vi "LSMcontroller_v63_3Dfocus.vi"() -> ()   [LabVIEW 2015] (continued)
                                w5034 = FALSE ("OK Button")
                                n2107 = property on="down" class="Bool (strict)"("Value"=w5034) -> ()  [unwired: 2 in, 2 out]
                                n2108 = property on="up" class="Bool (strict)"("Value"=w5034) -> ()  [unwired: 2 in, 2 out]
                                n2109 = property on="right" class="Bool (strict)"("Value"=w5034) -> ()  [unwired: 2 in, 2 out]
                                n2110 = property on="left" class="Bool (strict)"("Value"=w5034) -> ()  [unwired: 2 in, 2 out]
                                n2111 = property on="upleft" class="Bool (strict)"("Value"=w5033) -> ()  [unwired: 2 in, 2 out]
                                n2112 = property on="upright" class="Bool (strict)"("Value"=w5033) -> ()  [unwired: 2 in, 2 out]
                                n2113 = property on="downleft" class="Bool (strict)"("Value"=w5033) -> ()  [unwired: 2 in, 2 out]
                                n2114 = property on="downright" class="Bool (strict)"("Value"=w5033) -> ()  [unwired: 2 in, 2 out]
                                }
                                }
                                }
                                }
                                }
                              }
                              n2115 = dll-call lib="phlib.dll" fn="_PH_GetCountRate@8" label="PH_GetCountRate"("devidx"=w4980, "channel"=1) -> (→"Ch1Rate":i32)  [unwired: 5 in, 2 out]
                              n2116 = local read "Stop"() -> (w4982:bool)
                              n2117 = local write "points recorded"(w4979) -> ()
                            }
                          }
                          frame #3 {
                            w5042 = FALSE ("Value (Signaling)")
                            n2118 = call "2pparameters.vi"("command"="get") -> ("params out"=w5036:T10)  [unwired: 1 in]
                            n2119 = Unbundle By Name(w5036) -> ("autoshutter"=w5037:bool)
                            n2120 = case shown="True" w5037 {
                              frame False {
                              }
                              frame True {
                                n2121 = call "shuttercontrol.vi"("command"="close") -> ()  [unwired: 1 in, 1 out]
                              }
                            }
                            n2122 = property on="Start" class="Bool (strict)"("Val(Sgnl)"=w5042) -> ()  [unwired: 2 in, 2 out]
                            n2123 = property on="Start" class="Bool (strict)"("Visible"=TRUE, "DisabledEnum"=T7."Enabled" ("Disabled")) -> ()  [unwired: 2 in, 2 out]
                            n2124 = property on="Stop" class="Bool (strict)"("Val(Sgnl)"=w5042) -> ()  [unwired: 2 in, 2 out]
                            n2125 = property on="Stop" class="Bool (strict)"("Visible"=FALSE, "DisabledEnum"=T7."Disabled" ("Disabled")) -> ()  [unwired: 2 in, 2 out]
                          }
                        }
                      }
                      frame Enabled {
                      }
                    }
                    n2126 = local write "64bit disabled"(TRUE ("64bit disabled")) -> ()
                  }
                }
              }
            }
          }
          event "avpp", "Angle ref", "xpixels ref", "Vx-min ref", "Vx-max ref", "ypixels ref", "Vy-min ref", "Vy-max ref", "ROI Type", "Sampling rate": Value Change {
            n2127 = event-data() -> ()  [unwired: 1 in, 6 out]
            n2128 = local read "avpp"() -> (w5061:i32)
            n2129 = local read "Angle ref"() -> (w5060:dbl)
            n2130 = local read "ROI Type"() -> (w5059:u16)
            n2131 = local read "xpixels ref"() -> (w5056:i32)
            n2132 = local read "Vx-min ref"() -> (w5055:dbl)
            n2133 = local read "Vx-max ref"() -> (w5054:dbl)
            n2134 = local read "ypixels ref"() -> (w5052:i32)
            n2135 = local read "Vy-min ref"() -> (w5053:dbl)
            n2136 = local read "Vy-max ref"() -> (w5049:dbl)
            n2137 = local read "Sampling rate"() -> (w5044:dbl)
            n2138 = local read "# of frames"() -> (w5048:i32)
            n2139 = local read "maxbufferAI"() -> (w5047:i32)
            n2140 = local read "Override AI buffer"() -> (w5045:bool)
            n2141 = call "2pparameters.vi"("command"="get") -> ("params out"=w5058:T10)  [unwired: 1 in]
            n2142 = Bundle By Name(cluster=w5058, "avpp"=w5061, "Angle Img"=w5060, "Xpixels Img"=w5056, "Vx-min Img"=w5055, "VX-max Img"=w5054, "Ypixels Img"=w5052, "Vy-min Img"=w5053, "Vy-max Img"=w5049, "srate"=w5044, "srate Img"=w5044, "measpoints"=w5048, "maxbufferAI"=w5047, "Drawing Mode"=w5059, "Vz-reset"=0.0, "AIoverride"=w5045) -> (w5050:T10)
            n2143 = call "2pparameters.vi"("Params in"=w5050, "command"="set") -> ()  [unwired: 1 out]
          }
          event "# of frames": Value Change {
            n2144 = event-data() -> ()  [unwired: 1 in, 6 out]
            n2145 = local read "Meastab"() -> (w5062:enum32{"X-Y Image", "Linescan", "Timetrace"})
            n2146 = case shown="\"X-Y Image\", Default" w5062 {
              frame "X-Y Image", Default {
                n2147 = local read "# of frames"() -> (w5063:i32)
                n2148 = call "2pparameters.vi"("command"="get") -> ("params out"=w5067:T10)  [unwired: 1 in]
                n2149 = Bundle By Name(cluster=w5067, "measpoints"=w5063) -> (w5064:T10)
                n2150 = call "2pparameters.vi"("Params in"=w5064, "command"="set") -> ()  [unwired: 1 out]
              }
              frame "Linescan" {
                n2151 = local read "srateAODOtt"() -> (w5077:dbl)
                n2152 = local read "# of frames"() -> (w5073:i32)
                n2153 = local read "refreshtime"() -> (w5079:dbl)
                n2154 = local read "bin"() -> (w5074:dbl)
                n2155 = call "tt_timeandsamples.vi"("bin"=w5074, "refreshtime"=w5079, "srateAODOtt"=w5077, "tot#ofsamples"=w5073) -> ("refreshrate"=w5076:dbl, "refreshbuffer"=w5075:i32, "timetracecycles"=w5072:i32)  [unwired: 5 in]
                n2156 = call "2pparameters.vi"("command"="get") -> ("params out"=w5069:T10)  [unwired: 1 in]
                n2157 = Bundle By Name(cluster=w5069, "measpoints"=w5073, "tt_cycles"=w5072, "refreshbuffer"=w5075, "refreshrate"=w5076) -> (w5071:T10)
                n2158 = Reciprocal(x=w5076) -> (1/x=w5078:dbl)
                n2159 = local write "refreshtime"(w5078) -> ()
                n2160 = call "2pparameters.vi"("Params in"=w5071, "command"="set") -> ()  [unwired: 1 out]
              }
              frame "Timetrace" {
                n2161 = local read "srateAODOtt"() -> (w5089:dbl)
                n2162 = local read "# of frames"() -> (w5085:i32)
                n2163 = local read "refreshtime"() -> (w5091:dbl)
                n2164 = local read "bin"() -> (w5086:dbl)
                n2165 = call "tt_timeandsamples.vi"("bin"=w5086, "refreshtime"=w5091, "srateAODOtt"=w5089, "tot#ofsamples"=w5085) -> ("refreshrate"=w5088:dbl, "refreshbuffer"=w5087:i32, "timetracecycles"=w5084:i32)  [unwired: 5 in]
                n2166 = call "2pparameters.vi"("command"="get") -> ("params out"=w5081:T10)  [unwired: 1 in]
                n2167 = Bundle By Name(cluster=w5081, "measpoints"=w5085, "tt_cycles"=w5084, "refreshbuffer"=w5087, "refreshrate"=w5088) -> (w5083:T10)
                n2168 = Reciprocal(x=w5088) -> (1/x=w5090:dbl)
                n2169 = local write "refreshtime"(w5090) -> ()
                n2170 = call "2pparameters.vi"("Params in"=w5083, "command"="set") -> ()  [unwired: 1 out]
              }
            }
          }
          event "srateAODOtt", "refreshtime", "Vx-ref", "Vy-ref", "Vx-min draw", "Vx-max draw", "Vy-min draw", "Vy-max draw", "bin": Value Change {
            n2171 = event-data() -> ()  [unwired: 1 in, 6 out]
            n2172 = local read "ypixels ref"() -> (w5123:i32)
            n2173 = local read "Vy-min draw"() -> (w5099:dbl)
            n2174 = local read "Vy-max draw"() -> (w5098:dbl)
            n2175 = local read "Vx-min draw"() -> (w5101:dbl)
            n2176 = local read "Vx-max draw"() -> (w5100:dbl)
            n2177 = local read "xpixels ref"() -> (w5097:i32)
            n2178 = local read "ROI Type"() -> (w5096:u16)
            n2179 = local read "Pel"() -> (w5095:dbl)
            n2180 = local read "srateAODOtt"() -> (w5105:dbl)
            n2181 = local read "# of frames"() -> (w5110:i32)
            n2182 = local read "refreshtime"() -> (w5103:dbl)
            n2183 = local read "bin"() -> (w5108:dbl)
            n2184 = local read "Override AI buffer"() -> (w5093:bool)
            n2185 = local read "finite samples"() -> (w5117:bool)
            n2186 = local read "srateAODOtt"() -> (w5092:dbl)
            n2187 = local read "srateAODOtt"() -> (w5111:dbl)
            n2188 = local read "continuous"() -> (w5116:bool)
            n2189 = local read "Angle ref"() -> (w5102:dbl)
            n2190 = local read "wavdet"() -> (w5118:bool)
            n2191 = local read "Vx-ref"() -> (w5113:dbl)
            n2192 = local read "Vy-ref"() -> (w5115:dbl)
            n2193 = local read "avpp"() -> (w5114:i32)
            n2194 = call "tt_timeandsamples.vi"("bin"=w5108, "refreshtime"=w5103, "srateAODOtt"=w5105, "tot#ofsamples"=w5110) -> ("refreshrate"=w5106:dbl, "refreshbuffer"=w5107:i32, "timetracecycles"=w5112:i32)  [unwired: 5 in]
            n2195 = local read "bin"() -> (w5109:dbl)
            n2196 = call "2pparameters.vi"("command"="get") -> ("params out"=w5121:T10)  [unwired: 1 in]
            n2197 = Bundle By Name(cluster=w5121, "Drawing Mode"=w5096, "measpoints"=w5110, "tt_cycles"=w5112, "refreshbuffer"=w5107, "refreshrate"=w5106, "Vx-ref"=w5113, "Vy-ref"=w5115, "srate"=w5092, "finite"=w5117, "cont"=w5116, "wavdet"=w5118, "avpp"=w5114, "srateAODO"=w5111, "bufferAI"=w5107, "bin"=w5109, "Angle Img"=w5102, "Vxminref"=w5101, "Vxmaxref"=w5100, "Vyminref"=w5099, "Vymaxref"=w5098, "Xpixels Img"=w5097, "Ypixels Img"=w5123, "Pel"=w5095, "Vz-reset"=0.0, "AIoverride"=w5093) -> (w5119:T10)
            n2198 = Reciprocal(x=w5106) -> (1/x=w5104:dbl)
            n2199 = local write "refreshtime"(w5104) -> ()
            n2200 = call "2pparameters.vi"("Params in"=w5119, "command"="set") -> ()  [unwired: 1 out]
          }
          event "Init": Value Change {
            # "Disabled for conversion to 64 bit"
            n2201 = event-data() -> ()  [unwired: 1 in, 6 out]
            n2202 = disable-structure shown="Disabled" {
              frame Disabled {
                n2203 = flat-sequence {
                  frame #0 {
                    n2204 = local read "Measurement"() -> (w5125:T4)
                    n2205 = case shown="\"Lifetime (scan)\", \"Lifetime (contour)\"" w5125 {
                      frame "X-Y-t movie", Default {
                      }
                      frame "Lifetime (point)" {
                        n2206 = stacked-sequence {
                          frame #0 {
                            n2207 = call "initialize.vi"("mode"=0) -> ()
                          }
                          frame #1 {
                            n2208 = call "calib.vi"() -> ()  [unwired: 1 in]
                          }
                        }
                      }
                      frame "Lifetime (scan)", "Lifetime (contour)" {
                        n2209 = stacked-sequence {
                          frame #0 {
                            n2210 = call "initialize.vi"("mode"=3) -> ()
                          }
                          frame #1 {
                            n2211 = call "calib.vi"() -> ()  [unwired: 1 in]
                          }
                        }
                      }
                    }
                  }
                  frame #1 {
                    n2212 = property on="Start" class="Bool (strict)"("Visible"=TRUE, "DisabledEnum"=T7."Enabled" ("Disabled")) -> ()  [unwired: 2 in, 2 out]
                    n2213 = property on="Init" class="Bool (strict)"("Visible"=FALSE, "DisabledEnum"=T7."Disabled and Grayed Out" ("Disabled"), "Value"=FALSE ("Init")) -> ()  [unwired: 2 in, 2 out]
                  }
                }
              }
              frame Enabled {
              }
            }
            n2214 = local write "64bit disabled"(TRUE ("64bit disabled")) -> ()
          }
          event "Measurement": Value Change {
            n2215 = event-data() -> ()  [unwired: 1 in, 5 out]
            n2216 = case shown="\"X-Y-t movie\"" "Measurement" {
              frame "X-Y-t movie" {
                w5135 = T7."Disabled" ("Disabled")
                w5134 = FALSE ("Visible")
                n2217 = call "2pparameters.vi"("command"="get") -> ("params out"=w5145:T10)  [unwired: 1 in]
                n2218 = local write "graphtab"(T5."image" ("graphtab")) -> ()
                n2219 = local write "Save tab"(enum32{"withsave", "withoutsave"}."withsave" ("Save tab")) -> ()
                n2220 = Bundle By Name(cluster=w5145, "type"="X-Y-t movie") -> (w5143:T10)
                n2221 = call "2pparameters.vi"("Params in"=w5143, "command"="set") -> ()  [unwired: 1 out]
                n2222 = property on="refreshtime" class="DigNum (strict)"("Visible"=FALSE, "DisabledEnum"=T7."Disabled and Grayed Out" ("Disabled")) -> ()  [unwired: 2 in, 2 out]
                n2223 = property on="ttt" class="Enum (strict)"("Visible"=FALSE) -> ()  [unwired: 2 in, 2 out]
                n2224 = property on="# of frames" class="DigNum (strict)"("DisabledEnum"=T7."Enabled" ("Disabled"), "Caption.Text"="# of frames") -> ()  [unwired: 2 in, 2 out]
                n2225 = property on="continuous" class="Bool (strict)"("Visible"=TRUE, "DisabledEnum"=T7."Enabled" ("Disabled")) -> ()  [unwired: 2 in, 2 out]
                n2226 = property on="finite samples" class="Bool (strict)"("Visible"=TRUE, "DisabledEnum"=T7."Enabled" ("Disabled")) -> ()  [unwired: 2 in, 2 out]
                n2227 = property on="avpp" class="DigNum (strict)"("Visible"=TRUE, "DisabledEnum"=T7."Enabled" ("Disabled")) -> ()  [unwired: 2 in, 2 out]
                n2228 = property on="srateAODOtt" class="DigNum (strict)"("Visible"=FALSE, "DisabledEnum"=T7."Disabled" ("Disabled")) -> ()  [unwired: 2 in, 2 out]
                n2229 = local write "save\ndata"(TRUE ("save\ndata")) -> ()
                n2230 = property on="finite samples" class="Bool (strict)"("Val(Sgnl)"=TRUE ("continuous for display")) -> ()  [unwired: 2 in, 2 out]
                n2231 = property on="continuous" class="Bool (strict)"("Value"=FALSE ("continuous for display")) -> ()  [unwired: 2 in, 2 out]
                n2232 = property on="Current Average" class="DigNum (strict)"("Visible"=TRUE, "DisabledEnum"=T7."Enabled" ("Disabled")) -> ()  [unwired: 2 in, 2 out]
                n2233 = property on="img_CH1" class="IntGraph (strict)"("ZScale.Maximum"=7.0 ("Z Scale.Range:Maximum")) -> ()  [unwired: 2 in, 2 out]
                n2234 = property on="Sampling rate" class="DigNum (strict)"("Visible"=TRUE, "DisabledEnum"=T7."Enabled" ("Disabled")) -> ()  [unwired: 2 in, 2 out]
                n2235 = property on="Pel" class="DigNum (strict)"("Visible"=w5134, "DisabledEnum"=w5135) -> ()  [unwired: 2 in, 2 out]
                n2236 = property on="bin" class="DigNum (strict)"("Visible"=w5134, "DisabledEnum"=w5135) -> ()  [unwired: 2 in, 2 out]
                "Meastab" <- enum32{"X-Y Image", "Linescan", "Timetrace"}."X-Y Image" ("Meastab")
                "Zscantab" <- enum32{"withzscan", "withoutzscan", "lifetime"}."withoutzscan" ("Zscantab")
              }
              frame "X-Y-Z stack" {
                w5167 = T7."Disabled" ("Disabled")
                w5166 = FALSE ("Visible")
                n2237 = call "2pparameters.vi"("command"="get") -> ("params out"=w5177:T10)  [unwired: 1 in]
                n2238 = call "2pparameters.vi"("command"="get") -> ("params out"=w5181:T10)  [unwired: 1 in]
                n2239 = Bundle By Name(cluster=w5177, "type"="X-Y-Z stack") -> (w5175:T10)
                n2240 = Unbundle By Name(w5181) -> ("motorref"=w5180:refnum<k7>)
                n2241 = call "2pparameters.vi"("Params in"=w5175, "command"="set") -> ()  [unwired: 1 out]
                n2242 = local write "Zscantab"(enum32{"withzscan", "withoutzscan", "lifetime"}."withzscan" ("Zscantab")) -> ()
                n2243 = local write "Meastab"(enum32{"X-Y Image", "Linescan", "Timetrace"}."X-Y Image" ("Meastab")) -> ()
                n2244 = invoke class="MG17Motor" method="GetPosition"(reference=w5180, "lChanID"=0, "pfPosition"=sgl 0.0) -> ("pfPosition"=w5192:sgl)  [unwired: 2 in, 4 out]
                n2245 = property on="refreshtime" class="DigNum (strict)"("Visible"=FALSE, "DisabledEnum"=T7."Disabled and Grayed Out" ("Disabled")) -> ()  [unwired: 2 in, 2 out]
                n2246 = property on="ttt" class="Enum (strict)"("Visible"=FALSE) -> ()  [unwired: 2 in, 2 out]
                n2247 = Multiply(x=w5192, y=1000.0) -> (x*y=w5191:dbl)
                n2248 = local write "Actual Z position"(w5191) -> ()
                n2249 = local write "Save tab"(enum32{"withsave", "withoutsave"}."withsave" ("Save tab")) -> ()
                n2250 = property on="finite samples" class="Bool (strict)"("Visible"=FALSE, "DisabledEnum"=T7."Disabled and Grayed Out" ("Disabled")) -> ()  [unwired: 2 in, 2 out]
                n2251 = property on="avpp" class="DigNum (strict)"("Visible"=TRUE, "DisabledEnum"=T7."Enabled" ("Disabled")) -> ()  [unwired: 2 in, 2 out]
                n2252 = property on="continuous" class="Bool (strict)"("Visible"=FALSE, "DisabledEnum"=T7."Disabled and Grayed Out" ("Disabled")) -> ()  [unwired: 2 in, 2 out]
                n2253 = property on="img_CH1" class="IntGraph (strict)"("ZScale.Maximum"=7.0 ("Z Scale.Range:Maximum")) -> ()  [unwired: 2 in, 2 out]
                n2254 = property on="srateAODOtt" class="DigNum (strict)"("Visible"=FALSE, "DisabledEnum"=T7."Disabled" ("Disabled")) -> ()  [unwired: 2 in, 2 out]
                n2255 = property on="Pel" class="DigNum (strict)"("Visible"=w5166, "DisabledEnum"=w5167) -> ()  [unwired: 2 in, 2 out]
                n2256 = property on="bin" class="DigNum (strict)"("Visible"=w5166, "DisabledEnum"=w5167) -> ()  [unwired: 2 in, 2 out]
                n2257 = property on="Current Average" class="DigNum (strict)"("Visible"=TRUE, "DisabledEnum"=T7."Enabled" ("Disabled")) -> ()  [unwired: 2 in, 2 out]
                n2258 = property on="# of frames" class="DigNum (strict)"("Caption.Text"="# of slices", "DisabledEnum"=T7."Disabled and Grayed Out" ("Disabled")) -> ()  [unwired: 2 in, 2 out]
                n2259 = local write "save\ndata"(TRUE ("save\ndata")) -> ()
                n2260 = property on="finite samples" class="Bool (strict)"("Val(Sgnl)"=TRUE ("continuous for display")) -> ()  [unwired: 2 in, 2 out]
                n2261 = property on="continuous" class="Bool (strict)"("Value"=FALSE ("continuous for display")) -> ()  [unwired: 2 in, 2 out]
                n2262 = property on="Sampling rate" class="DigNum (strict)"("Visible"=TRUE, "DisabledEnum"=T7."Enabled" ("Disabled")) -> ()  [unwired: 2 in, 2 out]
              }
              frame "X-Y-Z-t movie" {
                w5206 = T7."Disabled" ("Disabled")
                w5205 = FALSE ("Visible")
                n2263 = property on="# of frames" class="DigNum (strict)"("DisabledEnum"=T7."Enabled" ("Disabled")) -> ()  [unwired: 2 in, 2 out]
                n2264 = property on="Current Average" class="DigNum (strict)"("Visible"=TRUE, "DisabledEnum"=T7."Enabled" ("Disabled")) -> ()  [unwired: 2 in, 2 out]
                n2265 = property on="avpp" class="DigNum (strict)"("Visible"=TRUE, "DisabledEnum"=T7."Enabled" ("Disabled")) -> ()  [unwired: 2 in, 2 out]
                n2266 = local write "Save tab"(enum32{"withsave", "withoutsave"}."withsave" ("Save tab")) -> ()
                n2267 = local write "Zscantab"(enum32{"withzscan", "withoutzscan", "lifetime"}."withzscan" ("Zscantab")) -> ()
                n2268 = local write "Meastab"(enum32{"X-Y Image", "Linescan", "Timetrace"}."X-Y Image" ("Meastab")) -> ()
                n2269 = property on="refreshtime" class="DigNum (strict)"("Visible"=FALSE, "DisabledEnum"=T7."Disabled and Grayed Out" ("Disabled")) -> ()  [unwired: 2 in, 2 out]
                n2270 = property on="ttt" class="Enum (strict)"("Visible"=FALSE) -> ()  [unwired: 2 in, 2 out]
                n2271 = call "2pparameters.vi"("command"="get") -> ("params out"=w5216:T10)  [unwired: 1 in]
                n2272 = Bundle By Name(cluster=w5216, "type"="X-Y-Z-t movie") -> (w5214:T10)
                n2273 = property on="continuous" class="Bool (strict)"("Visible"=TRUE, "DisabledEnum"=T7."Enabled" ("Disabled")) -> ()  [unwired: 2 in, 2 out]
                n2274 = property on="finite samples" class="Bool (strict)"("Visible"=TRUE, "DisabledEnum"=T7."Enabled" ("Disabled")) -> ()  [unwired: 2 in, 2 out]
                n2275 = call "2pparameters.vi"("Params in"=w5214, "command"="set") -> ()  [unwired: 1 out]
                n2276 = property on="srateAODOtt" class="DigNum (strict)"("Visible"=FALSE, "DisabledEnum"=T7."Disabled" ("Disabled")) -> ()  [unwired: 2 in, 2 out]
                n2277 = local write "save\ndata"(TRUE ("save\ndata")) -> ()
                n2278 = property on="img_CH1" class="IntGraph (strict)"("ZScale.Maximum"=7.0 ("Z Scale.Range:Maximum")) -> ()  [unwired: 2 in, 2 out]
                n2279 = property on="continuous" class="Bool (strict)"("Value"=FALSE ("continuous for display")) -> ()  [unwired: 2 in, 2 out]
                n2280 = property on="finite samples" class="Bool (strict)"("Value"=TRUE ("continuous for display")) -> ()  [unwired: 2 in, 2 out]
                n2281 = property on="Sampling rate" class="DigNum (strict)"("Visible"=TRUE, "DisabledEnum"=T7."Enabled" ("Disabled")) -> ()  [unwired: 2 in, 2 out]
                n2282 = property on="Pel" class="DigNum (strict)"("Visible"=w5205, "DisabledEnum"=w5206) -> ()  [unwired: 2 in, 2 out]
                n2283 = property on="bin" class="DigNum (strict)"("Visible"=w5205, "DisabledEnum"=w5206) -> ()  [unwired: 2 in, 2 out]
              }
              frame "linescan" {
                w5236 = T7."Enabled" ("Disabled")
                w5235 = TRUE ("Visible")
                w5238 = T7."Enabled" ("Disabled")
                w5237 = TRUE ("Visible")
                n2284 = local write "Meastab"(enum32{"X-Y Image", "Linescan", "Timetrace"}."Linescan" ("Meastab")) -> ()
                n2285 = property on="Current Average" class="DigNum (strict)"("Visible"=TRUE, "DisabledEnum"=T7."Enabled" ("Disabled")) -> ()  [unwired: 2 in, 2 out]
                n2286 = local write "Save tab"(enum32{"withsave", "withoutsave"}."withsave" ("Save tab")) -> ()
                n2287 = local write "Zscantab"(enum32{"withzscan", "withoutzscan", "lifetime"}."withoutzscan" ("Zscantab")) -> ()
                n2288 = property on="refreshtime" class="DigNum (strict)"("Visible"=FALSE, "DisabledEnum"=T7."Disabled and Grayed Out" ("Disabled")) -> ()  [unwired: 2 in, 2 out]
                n2289 = property on="continuous" class="Bool (strict)"("Value"=FALSE ("continuous for display")) -> ()  [unwired: 2 in, 2 out]
                n2290 = property on="finite samples" class="Bool (strict)"("Value"=TRUE ("continuous for display")) -> ()  [unwired: 2 in, 2 out]
                n2291 = property on="ttt" class="Enum (strict)"("Visible"=FALSE) -> ()  [unwired: 2 in, 2 out]
                n2292 = local write "save\ndata"(TRUE ("save\ndata")) -> ()
                n2293 = call "2pparameters.vi"("command"="get") -> ("params out"=w5247:T10)  [unwired: 1 in]
                n2294 = Bundle By Name(cluster=w5247, "type"="linescan") -> (w5245:T10)
                n2295 = property on="# of frames" class="DigNum (strict)"("DisabledEnum"=T7."Enabled" ("Disabled"), "Caption.Text"="# of lines") -> ()  [unwired: 2 in, 2 out]
                n2296 = property on="continuous" class="Bool (strict)"("Visible"=TRUE, "DisabledEnum"=T7."Enabled" ("Disabled")) -> ()  [unwired: 2 in, 2 out]
                n2297 = property on="avpp" class="DigNum (strict)"("Visible"=TRUE, "DisabledEnum"=T7."Enabled" ("Disabled")) -> ()  [unwired: 2 in, 2 out]
                n2298 = property on="finite samples" class="Bool (strict)"("Visible"=TRUE, "DisabledEnum"=T7."Enabled" ("Disabled")) -> ()  [unwired: 2 in, 2 out]
                n2299 = property on="srateAODOtt" class="DigNum (strict)"("Visible"=TRUE, "DisabledEnum"=T7."Enabled" ("Disabled")) -> ()  [unwired: 2 in, 2 out]
                n2300 = call "2pparameters.vi"("Params in"=w5245, "command"="set") -> ()  [unwired: 1 out]
                n2301 = property on="Pel" class="DigNum (strict)"("Visible"=w5237, "DisabledEnum"=w5238) -> ()  [unwired: 2 in, 2 out]
                n2302 = property on="bin" class="DigNum (strict)"("Visible"=w5237, "DisabledEnum"=w5238) -> ()  [unwired: 2 in, 2 out]
                n2303 = property on="Sampling rate" class="DigNum (strict)"("Visible"=FALSE, "DisabledEnum"=T7."Disabled" ("Disabled")) -> ()  [unwired: 2 in, 2 out]
                n2304 = property on="Pel" class="DigNum (strict)"("Visible"=w5235, "DisabledEnum"=w5236) -> ()  [unwired: 2 in, 2 out]
                n2305 = property on="bin" class="DigNum (strict)"("Visible"=w5235, "DisabledEnum"=w5236) -> ()  [unwired: 2 in, 2 out]
              }
              frame "Timetrace" {
                w5268 = T7."Enabled" ("Disabled")
                w5267 = TRUE ("Visible")
                n2306 = call "2pparameters.vi"("command"="get") -> ("params out"=w5273:T10)  [unwired: 1 in]
                n2307 = local write "Meastab"(enum32{"X-Y Image", "Linescan", "Timetrace"}."Timetrace" ("Meastab")) -> ()
                n2308 = Unbundle By Name(w5273) -> ("Angle draw"=w5275:dbl)
                n2309 = local write "Zscantab"(enum32{"withzscan", "withoutzscan", "lifetime"}."withoutzscan" ("Zscantab")) -> ()
                n2310 = property on="# of frames" class="DigNum (strict)"("DisabledEnum"=T7."Enabled" ("Disabled"), "Caption.Text"="# of samples") -> ()  [unwired: 2 in, 2 out]
                n2311 = property on="refreshtime" class="DigNum (strict)"("Visible"=TRUE, "DisabledEnum"=T7."Enabled" ("Disabled")) -> ()  [unwired: 2 in, 2 out]
                n2312 = property on="avpp" class="DigNum (strict)"("Visible"=FALSE, "DisabledEnum"=T7."Disabled and Grayed Out" ("Disabled")) -> ()  [unwired: 2 in, 2 out]
                n2313 = property on="Current Average" class="DigNum (strict)"("Visible"=FALSE, "DisabledEnum"=T7."Disabled and Grayed Out" ("Disabled")) -> ()  [unwired: 2 in, 2 out]
                n2314 = local write "Angle drawing"(w5275) -> ()
                n2315 = property on="ttt" class="Enum (strict)"("Visible"=TRUE) -> ()  [unwired: 2 in, 2 out]
                n2316 = property on="continuous" class="Bool (strict)"("Visible"=TRUE, "DisabledEnum"=T7."Enabled" ("Disabled")) -> ()  [unwired: 2 in, 2 out]
                n2317 = property on="finite samples" class="Bool (strict)"("Visible"=TRUE, "DisabledEnum"=T7."Enabled" ("Disabled")) -> ()  [unwired: 2 in, 2 out]
                n2318 = local write "save\ndata"(TRUE ("save\ndata")) -> ()
                n2319 = property on="finite samples" class="Bool (strict)"("Val(Sgnl)"=TRUE ("continuous for display")) -> ()  [unwired: 2 in, 2 out]
                n2320 = property on="continuous" class="Bool (strict)"("Value"=FALSE ("continuous for display")) -> ()  [unwired: 2 in, 2 out]
                n2321 = local write "Save tab"(enum32{"withsave", "withoutsave"}."withsave" ("Save tab")) -> ()
                n2322 = property on="srateAODOtt" class="DigNum (strict)"("Visible"=TRUE, "DisabledEnum"=T7."Enabled" ("Disabled")) -> ()  [unwired: 2 in, 2 out]
                n2323 = call "2pparameters.vi"("command"="get") -> ("params out"=w5280:T10)  [unwired: 1 in]
                n2324 = Bundle By Name(cluster=w5280, "type"="Timetrace") -> (w5278:T10)
                n2325 = property on="Sampling rate" class="DigNum (strict)"("Visible"=FALSE, "DisabledEnum"=T7."Disabled" ("Disabled")) -> ()  [unwired: 2 in, 2 out]
                n2326 = property on="Pel" class="DigNum (strict)"("Visible"=w5267, "DisabledEnum"=w5268) -> ()  [unwired: 2 in, 2 out]
                n2327 = property on="bin" class="DigNum (strict)"("Visible"=w5267, "DisabledEnum"=w5268) -> ()  [unwired: 2 in, 2 out]
                n2328 = call "2pparameters.vi"("Params in"=w5278, "command"="set") -> ()  [unwired: 1 out]
              }
              frame "Lifetime (point)" {
                w5301 = T7."Enabled" ("Disabled")
                w5300 = TRUE ("Visible")
                n2329 = property on="Pel" class="DigNum (strict)"("Visible"=w5300, "DisabledEnum"=w5301) -> ()  [unwired: 2 in, 2 out]
                n2330 = property on="bin" class="DigNum (strict)"("Visible"=w5300, "DisabledEnum"=w5301) -> ()  [unwired: 2 in, 2 out]
                n2331 = property on="ttt" class="Enum (strict)"("Visible"=FALSE) -> ()  [unwired: 2 in, 2 out]
                n2332 = local write "Zscantab"(enum32{"withzscan", "withoutzscan", "lifetime"}."lifetime" ("Zscantab")) -> ()
                n2333 = local write "graphtab"(T5."Lifetime" ("graphtab")) -> ()
                n2334 = local write "Meastab"(enum32{"X-Y Image", "Linescan", "Timetrace"}."Timetrace" ("Meastab")) -> ()
                n2335 = call "lifetimeparameters.vi"("command"="get") -> ("Params out"=w5308:T19)  [unwired: 1 in]
                n2336 = Unbundle By Name(w5308) -> ("initialized"=w5309:bool)
                n2337 = property on="srateAODOtt" class="DigNum (strict)"("Visible"=TRUE, "DisabledEnum"=T7."Enabled" ("Disabled")) -> ()  [unwired: 2 in, 2 out]
                n2338 = case shown="False" w5309 {
                  frame False {
                    n2339 = property on="Init" class="Bool (strict)"("Visible"=TRUE, "DisabledEnum"=T7."Enabled" ("Disabled")) -> ()  [unwired: 2 in, 2 out]
                    n2340 = property on="Start" class="Bool (strict)"("Visible"=FALSE, "DisabledEnum"=T7."Disabled and Grayed Out" ("Disabled")) -> ()  [unwired: 2 in, 2 out]
                  }
                  frame True {
                  }
                }
                n2341 = property on="Sampling rate" class="DigNum (strict)"("Visible"=FALSE, "DisabledEnum"=T7."Disabled" ("Disabled")) -> ()  [unwired: 2 in, 2 out]
              }
              frame "Lifetime (scan)" {
                w5318 = T7."Disabled" ("Disabled")
                w5317 = FALSE ("Visible")
                n2342 = call "lifetimeparameters.vi"("command"="get") -> ("Params out"=w5330:T19)  [unwired: 1 in]
                n2343 = local write "graphtab"(T5."image" ("graphtab")) -> ()
                n2344 = local write "Save tab"(enum32{"withsave", "withoutsave"}."withsave" ("Save tab")) -> ()
                n2345 = local write "Meastab"(enum32{"X-Y Image", "Linescan", "Timetrace"}."X-Y Image" ("Meastab")) -> ()
                n2346 = local write "Zscantab"(enum32{"withzscan", "withoutzscan", "lifetime"}."lifetime" ("Zscantab")) -> ()
                n2347 = Unbundle By Name(w5330) -> ("initialized"=w5329:bool)
                n2348 = property on="ttt" class="Enum (strict)"("Visible"=FALSE) -> ()  [unwired: 2 in, 2 out]
                n2349 = property on="refreshtime" class="DigNum (strict)"("Visible"=FALSE, "DisabledEnum"=T7."Disabled and Grayed Out" ("Disabled")) -> ()  [unwired: 2 in, 2 out]
                n2350 = property on="Pel" class="DigNum (strict)"("Visible"=w5317, "DisabledEnum"=w5318) -> ()  [unwired: 2 in, 2 out]
                n2351 = property on="bin" class="DigNum (strict)"("Visible"=w5317, "DisabledEnum"=w5318) -> ()  [unwired: 2 in, 2 out]
                n2352 = property on="save data" class="Bool (strict)"("Visible"=TRUE, "DisabledEnum"=T7."Enabled" ("Disabled"), "Value"=TRUE ("Visible")) -> ()  [unwired: 2 in, 2 out]
                n2353 = case shown="False" w5329 {
                  frame False {
                    n2354 = property on="Init" class="Bool (strict)"("Visible"=TRUE, "DisabledEnum"=T7."Enabled" ("Disabled")) -> ()  [unwired: 2 in, 2 out]
                    n2355 = property on="Start" class="Bool (strict)"("Visible"=FALSE, "DisabledEnum"=T7."Disabled and Grayed Out" ("Disabled")) -> ()  [unwired: 2 in, 2 out]
                  }
                  frame True {
                  }
                }
                n2356 = call "2pparameters.vi"("command"="get") -> ("params out"=w5335:T10)  [unwired: 1 in]
                n2357 = property on="continuous" class="Bool (strict)"("Visible"=TRUE, "DisabledEnum"=T7."Disabled and Grayed Out" ("Disabled")) -> ()  [unwired: 2 in, 2 out]
                n2358 = property on="finite samples" class="Bool (strict)"("Visible"=TRUE, "DisabledEnum"=T7."Enabled" ("Disabled")) -> ()  [unwired: 2 in, 2 out]
                n2359 = Bundle By Name(cluster=w5335, "type"="Lifetime (scan)") -> (w5333:T10)
                n2360 = call "2pparameters.vi"("Params in"=w5333, "command"="set") -> ()  [unwired: 1 out]
                n2361 = property on="finite samples" class="Bool (strict)"("Val(Sgnl)"=TRUE ("continuous for display")) -> ()  [unwired: 2 in, 2 out]
                n2362 = property on="continuous" class="Bool (strict)"("Value"=FALSE ("continuous for display")) -> ()  [unwired: 2 in, 2 out]
                n2363 = property on="srateAODOtt" class="DigNum (strict)"("Visible"=FALSE, "DisabledEnum"=T7."Disabled" ("Disabled")) -> ()  [unwired: 2 in, 2 out]
                n2364 = property on="# of frames" class="DigNum (strict)"("DisabledEnum"=T7."Enabled" ("Disabled"), "Caption.Text"="# of frames") -> ()  [unwired: 2 in, 2 out]
                n2365 = property on="img_CH1" class="IntGraph (strict)"("ZScale.Maximum"=12.5 ("Z Scale.Range:Maximum")) -> ()  [unwired: 2 in, 2 out]
                n2366 = property on="Current Average" class="DigNum (strict)"("Visible"=TRUE, "DisabledEnum"=T7."Enabled" ("Disabled")) -> ()  [unwired: 2 in, 2 out]
                n2367 = property on="Sampling rate" class="DigNum (strict)"("Visible"=TRUE, "DisabledEnum"=T7."Enabled" ("Disabled")) -> ()  [unwired: 2 in, 2 out]
                n2368 = property on="avpp" class="DigNum (strict)"("Visible"=TRUE, "DisabledEnum"=T7."Enabled" ("Disabled")) -> ()  [unwired: 2 in, 2 out]
              }
              frame "Lifetime (contour)" {
                w5359 = T7."Enabled" ("Disabled")
                w5358 = TRUE ("Visible")
                n2369 = call "2pparameters.vi"("command"="get") -> ("params out"=w5366:T10)  [unwired: 1 in]
                n2370 = property on="# of frames" class="DigNum (strict)"("DisabledEnum"=T7."Enabled" ("Disabled"), "Caption.Text"="# of samples") -> ()  [unwired: 2 in, 2 out]
                n2371 = property on="refreshtime" class="DigNum (strict)"("Visible"=TRUE, "DisabledEnum"=T7."Enabled" ("Disabled")) -> ()  [unwired: 2 in, 2 out]
                n2372 = Unbundle By Name(w5366) -> ("Angle draw"=w5368:dbl)
                n2373 = property on="avpp" class="DigNum (strict)"("Visible"=FALSE, "DisabledEnum"=T7."Disabled and Grayed Out" ("Disabled")) -> ()  [unwired: 2 in, 2 out]
                n2374 = property on="Current Average" class="DigNum (strict)"("Visible"=FALSE, "DisabledEnum"=T7."Disabled and Grayed Out" ("Disabled")) -> ()  [unwired: 2 in, 2 out]
                n2375 = local write "Angle drawing"(w5368) -> ()
                n2376 = local write "Save tab"(enum32{"withsave", "withoutsave"}."withsave" ("Save tab")) -> ()
                n2377 = local write "Zscantab"(enum32{"withzscan", "withoutzscan", "lifetime"}."lifetime" ("Zscantab")) -> ()
                n2378 = local write "graphtab"(T5."Lifetime" ("graphtab")) -> ()
                n2379 = local write "Meastab"(enum32{"X-Y Image", "Linescan", "Timetrace"}."Timetrace" ("Meastab")) -> ()
                n2380 = property on="ttt" class="Enum (strict)"("Visible"=TRUE) -> ()  [unwired: 2 in, 2 out]
                n2381 = call "lifetimeparameters.vi"("command"="get") -> ("Params out"=w5390:T19)  [unwired: 1 in]
                n2382 = property on="finite samples" class="Bool (strict)"("Val(Sgnl)"=TRUE ("continuous for display")) -> ()  [unwired: 2 in, 2 out]
                n2383 = local write "save\ndata"(TRUE ("save\ndata")) -> ()
                n2384 = Unbundle By Name(w5390) -> ("initialized"=w5391:bool)
                n2385 = property on="continuous" class="Bool (strict)"("Visible"=TRUE, "DisabledEnum"=T7."Enabled" ("Disabled")) -> ()  [unwired: 2 in, 2 out]
                n2386 = property on="finite samples" class="Bool (strict)"("Visible"=TRUE, "DisabledEnum"=T7."Enabled" ("Disabled")) -> ()  [unwired: 2 in, 2 out]
                n2387 = property on="Pel" class="DigNum (strict)"("Visible"=w5358, "DisabledEnum"=w5359) -> ()  [unwired: 2 in, 2 out]
                n2388 = property on="bin" class="DigNum (strict)"("Visible"=w5358, "DisabledEnum"=w5359) -> ()  [unwired: 2 in, 2 out]
                n2389 = property on="continuous" class="Bool (strict)"("Value"=FALSE ("continuous for display")) -> ()  [unwired: 2 in, 2 out]
                n2390 = case shown="False" w5391 {
                  frame False {
                    n2391 = property on="Init" class="Bool (strict)"("Visible"=TRUE, "DisabledEnum"=T7."Enabled" ("Disabled")) -> ()  [unwired: 2 in, 2 out]
                    n2392 = property on="Start" class="Bool (strict)"("Visible"=FALSE, "DisabledEnum"=T7."Disabled and Grayed Out" ("Disabled")) -> ()  [unwired: 2 in, 2 out]
                  }
                  frame True {
                  }
                }
                n2393 = property on="srateAODOtt" class="DigNum (strict)"("Visible"=TRUE, "DisabledEnum"=T7."Enabled" ("Disabled")) -> ()  [unwired: 2 in, 2 out]
                n2394 = call "2pparameters.vi"("command"="get") -> ("params out"=w5370:T10)  [unwired: 1 in]
                n2395 = Bundle By Name(cluster=w5370, "type"="Timetrace") -> (w5364:T10)
                n2396 = call "2pparameters.vi"("Params in"=w5364, "command"="set") -> ()  [unwired: 1 out]
                n2397 = property on="Sampling rate" class="DigNum (strict)"("Visible"=FALSE, "DisabledEnum"=T7."Disabled" ("Disabled")) -> ()  [unwired: 2 in, 2 out]
              }
            }
          }
          event "Laserpower \n(%)": Value Change {
            n2398 = event-data() -> ("OldVal"=w5399:dbl, "NewVal"=w5400:dbl)  [unwired: 1 in, 4 out]
            n2399 = Not Equal?(x=w5399, y=w5400) -> (x != y?=w5401:bool)
            n2400 = case shown="True" w5401 {
              tunnel: w5400 -> [_ w5403]
              frame False {
              }
              frame True {
                n2401 = local read "wavelength(nm)"() -> (w5404:dbl)
                n2402 = call "configuration.vi"("command"="get") -> ("config out"=w5408:T11)  [unwired: 2 in, 1 out]
                n2403 = call "pockelscellcalibration.vi"("l"=w5404, "T"=w5403) -> ("Vout"=w5402:dbl)
                n2404 = Unbundle By Name(w5408) -> ("Vto2P"=w5407:i32, "AOlines"=w5406:tag[])
                n2405 = property on="lpow" class="DigNum (strict)"("Value"=w5403) -> ()  [unwired: 2 in, 2 out]
                n2406 = local write "Vpockels"(w5402) -> ()
                n2407 = Index Array(array=w5406, index=w5407) -> (element=w5405:tag)
                n2408 = call-poly <vilib>:"DAQmx Create Virtual Channel.vi"("physical channels"=w5405) -> ("task out"=w5411:refnum<k21>, "error out"=w5410:errorcluster)  [unwired: 13 in]
                n2409 = call-poly <vilib>:"DAQmx Write.vi"("task/channels in"=w5411, "data"=w5402, "error in"=w5410) -> ("task out"=w5412:refnum<k21>, "error out"=w5413:errorcluster)  [unwired: 10 in, 1 out]
                n2410 = call <vilib>:"DAQmx Start Task.vi"("task/channels in"=w5412, "error in"=w5413) -> ("task out"=w5414:refnum<k21>, "error out"=w5415:errorcluster)  [unwired: 12 in]
                n2411 = call <vilib>:"DAQmx Stop Task.vi"("task/channels in"=w5414, "error in"=w5415) -> ("task out"=w5416:refnum<k21>, "error out"=w5417:errorcluster)  [unwired: 12 in]
                n2412 = call <vilib>:"DAQmx Clear Task.vi"("task in"=w5416, "error in"=w5417) -> ()  [unwired: 13 in, 1 out]
              }
            }
          }
          event "lpow": Value Change {
            n2413 = event-data() -> ("OldVal"=w5418:dbl, "NewVal"=w5419:dbl)  [unwired: 1 in, 4 out]
            n2414 = Not Equal?(x=w5418, y=w5419) -> (x != y?=w5420:bool)
            n2415 = case shown="True" w5420 {
              tunnel: w5419 -> [_ w5423]
              frame False {
              }
              frame True {
                n2416 = local read "wavelength(nm)"() -> (w5422:dbl)
                n2417 = call "pockelscellcalibration.vi"("l"=w5422, "T"=w5423) -> ("Vout"=w5421:dbl)
                n2418 = call "configuration.vi"("command"="get") -> ("config out"=w5427:T11)  [unwired: 2 in, 1 out]
                n2419 = Unbundle By Name(w5427) -> ("Vto2P"=w5426:i32, "AOlines"=w5425:tag[])
                n2420 = local write "Vpockels"(w5421) -> ()
                n2421 = property on="Laserpower \n(%)" class="Slide (strict)"("Value"=w5423) -> ()  [unwired: 2 in, 2 out]
                n2422 = Index Array(array=w5425, index=w5426) -> (element=w5424:tag)
                n2423 = call-poly <vilib>:"DAQmx Create Virtual Channel.vi"("physical channels"=w5424) -> ("task out"=w5430:refnum<k21>, "error out"=w5429:errorcluster)  [unwired: 13 in]
                n2424 = call-poly <vilib>:"DAQmx Write.vi"("task/channels in"=w5430, "data"=w5421, "error in"=w5429) -> ("task out"=w5431:refnum<k21>, "error out"=w5432:errorcluster)  [unwired: 10 in, 1 out]
                n2425 = call <vilib>:"DAQmx Start Task.vi"("task/channels in"=w5431, "error in"=w5432) -> ("task out"=w5433:refnum<k21>, "error out"=w5434:errorcluster)  [unwired: 12 in]
                n2426 = call <vilib>:"DAQmx Stop Task.vi"("task/channels in"=w5433, "error in"=w5434) -> ("task out"=w5435:refnum<k21>, "error out"=w5436:errorcluster)  [unwired: 12 in]
                n2427 = call <vilib>:"DAQmx Clear Task.vi"("task in"=w5435, "error in"=w5436) -> ()  [unwired: 13 in, 1 out]
              }
            }
          }
          event "sealtest": Value Change {
            n2428 = event-data() -> ()  [unwired: 1 in, 6 out]
            n2429 = case shown="True" "sealtest" {
              frame False {
              }
              frame True {
                n2430 = stacked-sequence {
                  seq-local: [w5438 _ _ _ _ _] -> [_ w5471 _ w5523 _ _]
                  frame #0 {
                    n2431 = stacked-sequence {
                      tunnel: [_ w5450 _] -> w5438
                      frame #0 {
                        n2432 = call "2pparameters.vi"("command"="get") -> ("params out"=w5443:T10)  [unwired: 1 in]
                        n2433 = Unbundle By Name(w5443) -> ("autoshutter"=w5444:bool)
                        n2434 = local read "OCchecked?"() -> (w5441:bool)
                        n2435 = call "sealtestwfparams.vi"("command"="set") -> ()  [unwired: 6 in, 1 out]
                        n2436 = case shown="False" w5441 {
                          frame False {
                            n2437 = One Button Dialog(message="Is the OC gain correct?", button name ("OK")="ok") -> (true=w5445:bool)
                            n2438 = local write "OCchecked?"(w5445) -> ()
                          }
                          frame True {
                          }
                        }
                        n2439 = case shown="True" w5444 {
                          frame False {
                          }
                          frame True {
                            n2440 = call "shuttercontrol.vi"("command"="close") -> ()  [unwired: 1 in, 1 out]
                          }
                        }
                        n2441 = call "allAI-temp.vi"("command"=enum16{"get", "set", "clear", "append"}."clear") -> ()  [unwired: 3 in, 2 out]
                      }
                      frame #1 {
                        n2442 = call "sealtestwfparams.vi"("command"="get") -> ("Params out"=w5456:T22)  [unwired: 6 in]
                        n2443 = Unbundle By Name(w5456) -> ("AO parameters"=w5454:T23)
                        n2444 = Index Array(array=w5454, index=0) -> (element=w5453:T24)
                        n2445 = call "generateRampedSquareWave_fromAOparameters.vi"("AO params"=w5453) -> ("Waveform"=w5449:waveform(dbl), "wflength"=w5450:i32)
                        n2446 = Build Array(w5449) -> (w5452:waveform(dbl)[])
                        n2447 = call "waveformssealtestbuffer.vi"("AO wf in"=w5452, "command"="set") -> ()  [unwired: 1 out]
                      }
                      frame #2 {
                        n2448 = local read "Vholding (mV)"() -> (w5459:sgl)
                        n2449 = local read "Current Clamp"() -> (w5465:bool)
                        n2450 = local read "Voltage Clamp"() -> (w5464:bool)
                        n2451 = local read "OCgain"() -> (w5460:sgl)
                        n2452 = local read "CC_ICgain"() -> (w5463:dbl)
                        n2453 = local read "holdon"() -> (w5458:bool)
                        n2454 = call "patchparameters.vi"("command"="get") -> ("Params out"=w5467:T13)  [unwired: 1 in]
                        n2455 = Bundle By Name(cluster=w5467, "VC"=w5464, "CC"=w5465, "CC_icg (pA/mv)"=w5463, "VC_icg (mV/mV)"=10.0, "OCG (mV/pA)"=w5460, "OVG (mV/mV)"=0.1, "Vhold (mV)"=w5459, "holdon"=w5458) -> (w5466:T13)
                        n2456 = call "patchparameters.vi"("Params in"=w5466, "command"="set") -> ()  [unwired: 1 out]
                      }
                    }
                  }
                  frame #1 {
                    w5470 = 2
                    n2457 = call "patchparameters.vi"("command"="get") -> ("Params out"=w5478:T13)  [unwired: 1 in]
                    n2458 = Unbundle By Name(w5478) -> ("holdon"=w5477:bool, "Vhold (mV)"=w5476:sgl, "CC_icg (pA/mv)"=w5484:sgl, "CC"=w5482:bool, "VC_icg (mV/mV)"=w5483:sgl)
                    n2459 = Select(t=w5484, s=w5482, f=w5483) -> (s? t:f=w5485:sgl)
                    n2460 = To Single Precision Float(number=0.001 ("y")) -> (single precision float=w5486:sgl)
                    n2461 = Compound Arithmetic op=MULTIPLY(w5476, w5485, w5486) -> (w5480:sgl)
                    n2462 = case shown="False" w5477 {
                      tunnel: w5480 -> [_ w5498]
                      tunnel: [0.0 w5498] -> w5473
                      frame False {
                      }
                      frame True {
                      }
                    }
                    n2463 = Greater Than 0?(x=w5470) -> (x > 0?=w5472:bool)
                    n2464 = case shown="True" w5472 {
                      tunnel: w5471 -> [_ w5487]
                      tunnel: w5470 -> [_ w5490]
                      frame False {
                      }
                      frame True {
                        n2465 = Initialize Array(sgl 0.0 ("element"), w5490, w5487) -> (w5488:sgl[][])
                        n2466 = call "allAI-temp.vi"("array in"=w5488, "command"=enum16{"get", "set", "clear", "append"}."set") -> ()  [unwired: 2 in, 2 out]
                      }
                    }
                    n2467 = flat-sequence {
                      tunnel: w5471 -> [w5494]
                      tunnel: w5471 -> [w5493]
                      tunnel: [w5493] -> w5475
                      tunnel: [w5492] -> w5474
                      tunnel: w5473 -> [w5492]
                      tunnel: w5475 -> [w5496]
                      tunnel: w5474 -> [w5495]
                      frame #0 {
                        n2468 = call "prepAI_sealtest.vi"("samples per channel"=w5494) -> ()  [unwired: 2 in]
                      }
                      frame #1 {
                        n2469 = call "prepAO_sealtest.vi"("Vhold"=w5495, "samples per channel"=w5496) -> ()  [unwired: 1 in]
                      }
                    }
                  }
                  frame #2 {
                    n2470 = stacked-sequence {
                      frame #0 {
                        n2471 = call "tempconfigAO.vi"("command"="get") -> ("Temp Config out"=w5502:T25)  [unwired: 1 in]
                        n2472 = Unbundle By Name(w5502) -> ("AO"=w5503:refnum<k21>[], "E_AO"=w5504:errorcluster[])
                        n2473 = for {
                          tunnel: w5503 -> [w5512] mode=indexing
                          tunnel: w5504 -> [w5511] mode=indexing
                          tunnel: [w5510] -> w5506 mode=indexing
                          tunnel: [w5509] -> w5507 mode=indexing
                          n2474 = call <vilib>:"DAQmx Start Task.vi"("task/channels in"=w5512, "error in"=w5511) -> ("task out"=w5510:refnum<k21>, "error out"=w5509:errorcluster)  [unwired: 12 in]
                        }
                        n2475 = call "tempconfigAO.vi"("command"="get") -> ("Temp Config out"=w5505:T25)  [unwired: 1 in]
                        n2476 = Bundle By Name(cluster=w5505, "AO"=w5506, "E_AO"=w5507) -> (w5508:T25)
                        n2477 = call "tempconfigAO.vi"("Temp Config in"=w5508, "command"="set") -> ()  [unwired: 1 out]
                      }
                      frame #1 {
                        n2478 = call "tempconfigAI.vi"("command"="get") -> ("Temp Config out"=w5514:T26)  [unwired: 1 in]
                        n2479 = Unbundle By Name(w5514) -> ("AI"=w5519:refnum<k21>, "E_AI"=w5520:errorcluster)
                        n2480 = call <vilib>:"DAQmx Start Task.vi"("task/channels in"=w5519, "error in"=w5520) -> ("task out"=w5521:refnum<k21>, "error out"=w5522:errorcluster)  [unwired: 12 in]
                        n2481 = call "tempconfigAI.vi"("command"="get") -> ("Temp Config out"=w5516:T26)  [unwired: 1 in]
                        n2482 = Bundle By Name(cluster=w5516, "AI"=w5521, "E_AI"=w5522) -> (w5518:T26)
                        n2483 = call "tempconfigAI.vi"("Temp Config in"=w5518, "command"="set") -> ()  [unwired: 1 out]
                      }
                    }
                  }
                  frame #3 {
                    n2484 = while {
                      tunnel: w5523 -> [w5524]
                      stop <- w5525 stop-if-true
                      n2485 = local read "sealtest"() -> (w5528:bool)
                      n2486 = Not(x=w5528) -> (.not. x?=w5527:bool)
                      n2487 = case shown="False" w5527 {
                        tunnel: w5524 -> [w5529 _]
                        frame False {
                          n2488 = stacked-sequence {
                            seq-local: [_ _ _ w5568 _ _] -> [_ _ _ _ w5624 _]
                            seq-local: [w5530 _ _ _ _ _] -> [_ w5539 _ w5561 w5613 w5644]
                            tunnel: w5529 -> [_ _ w5547 _ w5612 _]
                            frame #0 {
                              n2489 = call "patchparameters.vi"("command"="get") -> ("Params out"=w5537:T13)  [unwired: 1 in]
                              n2490 = local read "Vholding (mV)"() -> (w5534:sgl)
                              n2491 = Unbundle By Name(w5537) -> ("Vhold (mV)"=w5533:sgl, "holdon"=w5536:bool)
                              n2492 = local read "holdon"() -> (w5535:bool)
                              n2493 = Not Equal?(x=w5534, y=w5533) -> (x != y?=w5532:bool)
                              n2494 = Not Equal?(x=w5536, y=w5535) -> (x != y?=w5531:bool)
                              n2495 = Or(x=w5532, y=w5531) -> (x .or. y?=w5530:bool)
                            }
                            frame #1 {
                              n2496 = case shown="True" w5539 {
                                frame False {
                                }
                                frame True {
                                n2497 = local read "Vholding (mV)"() -> (w5542:sgl)
                                n2498 = local read "holdon"() -> (w5540:bool)
                                n2499 = call "patchparameters.vi"("command"="get") -> ("Params out"=w5543:T13)  [unwired: 1 in]
                                n2500 = Bundle By Name(cluster=w5543, "Vhold (mV)"=w5542, "holdon"=w5540) -> (w5541:T13)
                                n2501 = call "patchparameters.vi"("Params in"=w5541, "command"="set") -> ()  [unwired: 1 out]
                                }
                              }
                            }
                            frame #2 {
                              n2502 = call "tempconfigAI.vi"("command"="get") -> ("Temp Config out"=w5557:T26)  [unwired: 1 in]
                              n2503 = Unbundle By Name(w5557) -> ("AI"=w5556:refnum<k21>, "E_AI"=w5555:errorcluster)
                              n2504 = call-poly <vilib>:"DAQmx Read.vi"("task/channels in"=w5556, "number of samples per channel"=w5547, "timeout"=10.0, "error in"=w5555) -> ("task out"=w5551:refnum<k21>, "data"=w5548:i16[][], "error out"=w5560:errorcluster)  [unwired: 9 in]
                              n2505 = call "tempconfigAI.vi"("command"="get") -> ("Temp Config out"=w5552:T26)  [unwired: 1 in]
                              n2506 = Bundle By Name(cluster=w5552, "AI"=w5551, "E_AI"=w5560) -> (w5559:T26)
                              n2507 = To Single Precision Float(number=w5548) -> (single precision float=w5550:sgl[][])
                              n2508 = call "tempconfigAI.vi"("Temp Config in"=w5559, "command"="set") -> ()  [unwired: 1 out]
                              n2509 = call "allAI-temp.vi"("array in"=w5550, "command"=enum16{"get", "set", "clear", "append"}."set") -> ()  [unwired: 2 in, 2 out]
                            }
                            frame #3 {
                              n2510 = case shown="True" w5561 {
                                frame False {
                                }
                                frame True {
                                n2511 = call "tempconfigAO.vi"("command"="get") -> ("Temp Config out"=w5601:T25)  [unwired: 1 in]
                                n2512 = Unbundle By Name(w5601) -> ("AO"=w5600:refnum<k21>[], "E_AO"=w5599:errorcluster[])
                                n2513 = call "tempconfigAI.vi"("command"="get") -> ("Temp Config out"=w5588:T26)  [unwired: 1 in]
                                n2514 = Unbundle By Name(w5588) -> ("AI"=w5589:refnum<k21>, "E_AI"=w5590:errorcluster)
                                n2515 = for {
                                tunnel: w5600 -> [w5605] mode=indexing
                                tunnel: w5599 -> [w5604] mode=indexing
                                tunnel: [w5603] -> w5595 mode=indexing
                                n2516 = call <vilib>:"DAQmx Stop Task.vi"("task/channels in"=w5605, "error in"=w5604) -> ("task out"=w5606:refnum<k21>, "error out"=w5607:errorcluster)  [unwired: 12 in]
                                n2517 = call <vilib>:"DAQmx Clear Task.vi"("task in"=w5606, "error in"=w5607) -> ("error out"=w5603:errorcluster)  [unwired: 13 in]
                                }
                                n2518 = call <vilib>:"DAQmx Stop Task.vi"("task/channels in"=w5589, "error in"=w5590) -> ("task out"=w5586:refnum<k21>, "error out"=w5585:errorcluster)  [unwired: 12 in]
                                n2519 = call <vilib>:"DAQmx Clear Task.vi"("task in"=w5586, "error in"=w5585) -> ("error out"=w5584:errorcluster)  [unwired: 13 in]
                                n2520 = call "tempconfigAO.vi"("command"="get") -> ("Temp Config out"=w5596:T25)  [unwired: 1 in]
                                n2521 = Bundle By Name(cluster=w5596, "E_AO"=w5595) -> (w5594:T25)
                                n2522 = call "tempconfigAI.vi"("command"="get") -> ("Temp Config out"=w5592:T26)  [unwired: 1 in]
                                n2523 = Bundle By Name(cluster=w5592, "E_AI"=w5584) -> (w5583:T26)
                                n2524 = call "tempconfigAO.vi"("Temp Config in"=w5594, "command"="set") -> ()  [unwired: 1 out]
                                n2525 = call "tempconfigAI.vi"("Temp Config in"=w5583, "command"="set") -> ()  [unwired: 1 out]
                                }
                              }
                              n2526 = call "allAI-temp.vi"("command"=enum16{"get", "set", "clear", "append"}."get") -> ("array out"=w5565:sgl[][])  [unwired: 3 in, 1 out]
                              n2527 = call "tempconfigAI.vi"("command"="get") -> ("Temp Config out"=w5578:T26)  [unwired: 1 in]
                              n2528 = call "tempconfigAI.vi"("command"="get") -> ("Temp Config out"=w5580:T26)  [unwired: 1 in]
                              n2529 = Unbundle By Name(w5578) -> ("header"=w5576:dbl[])
                              n2530 = Unbundle By Name(w5580) -> ("header"=w5582:dbl[])
                              n2531 = Index Array(array=w5565, index (row) #1=1 ("index (row)"), index (row) #2=0 ("index (row)")) -> (element #1=w5563:sgl[], element #2=w5562:sgl[])  [unwired: 2 in]
                              n2532 = local read "OCgain"() -> (w5570:sgl)
                              n2533 = call "Unscaledtoscaled.vi"("Unscaled Data"=w5563, "Header Information"=w5576) -> ("Array"=w5575:sgl[])  [unwired: 1 in]
                              n2534 = call "Unscaledtoscaled.vi"("Unscaled Data"=w5562, "Header Information"=w5582) -> ("Array"=w5579:sgl[])  [unwired: 1 in]
                              n2535 = Multiply(x=w5575, y=0.1) -> (x*y=w5572:dbl[])
                              n2536 = Divide(x=w5579, y=w5570) -> (x/y=w5571:sgl[])
                              n2537 = Build Array(w5572, w5571) -> (w5574:dbl[][])
                              n2538 = Multiply(x=w5574, y=1000.0) -> (x*y=w5568:dbl[][])
                              "Patch readout" <- w5568
                            }
                            frame #4 {
                              n2539 = case shown="True" w5613 {
                                tunnel: w5612 -> [_ w5625]
                                frame False {
                                }
                                frame True {
                                n2540 = call "patchparameters.vi"("command"="get") -> ("Params out"=w5629:T13)  [unwired: 1 in]
                                n2541 = Unbundle By Name(w5629) -> ("holdon"=w5628:bool, "Vhold (mV)"=w5627:sgl, "CC_icg (pA/mv)"=w5635:sgl, "CC"=w5633:bool, "VC_icg (mV/mV)"=w5634:sgl)
                                n2542 = Select(t=w5635, s=w5633, f=w5634) -> (s? t:f=w5636:sgl)
                                n2543 = To Single Precision Float(number=0.001 ("y")) -> (single precision float=w5637:sgl)
                                n2544 = Compound Arithmetic op=MULTIPLY(w5627, w5636, w5637) -> (w5631:sgl)
                                n2545 = case shown="True" w5628 {
                                tunnel: w5631 -> [_ w5642]
                                tunnel: [0.0 w5642] -> w5626
                                frame False {
                                }
                                frame True {
                                }
                                }
                                n2546 = flat-sequence {
                                tunnel: w5625 -> [w5638]
                                tunnel: w5626 -> [w5640]
                                tunnel: w5625 -> [w5639]
                                frame #0 {
                                n2547 = call "prepAI_sealtest.vi"("samples per channel"=w5638) -> ()  [unwired: 2 in]
                                }
                                frame #1 {
                                n2548 = call "prepAO_sealtest.vi"("Vhold"=w5640, "samples per channel"=w5639) -> ()  [unwired: 1 in]
                                }
                                }
                                }
                              }
                              n2549 = call "sealtestwfparams.vi"("command"="get") -> ("Params out"=w5618:T22)  [unwired: 6 in]
                              n2550 = Unbundle By Name(w5618) -> ("AO parameters"=w5619:T23)
                              n2551 = Index Array(array=w5619, index=0) -> (element=w5621:T24)
                              n2552 = Unbundle By Name(w5621) -> ("Cycles"=w5616:dbl, "Start amplitude (V)"=w5615:dbl, "Sampling frequency (Hz)"=w5614:dbl)
                              n2553 = local read "fitpoints"() -> (w5622:dbl)
                              n2554 = script code="V=data(1,:);\nI=data(2,:);\ntres=mean(V);\nspc=(nsamp./ncyc);\nV=V(spc+1:end-spc);\nI=I(spc+1:end-spc);\ndV=mean(V(V>tres))-mean(V(V<tres))\nIcyc=reshape(I,[spc ncyc-2]);\nIcyc=Icyc';\nIcyc=mean(Icyc,1);\ndIss=mean(Icyc(floor(spc*0.15):floor(spc/2)-2))-mean(Icyc(spc*0.65:spc-2))\nRm=dV*1e3/dIss;\n[maxi,ind]=max(Icyc);\nIfit=Icyc(ind+1:ind+1+points-1)-0.5*(mean(Icyc(floor(spc*0.15):floor(spc/2)-2))+mean(Icyc(spc*0.65:spc-2)))\nt=(3:points-1+3)./srate*1000;\nt=t';\nIfit=Ifit';\nc=fit(t,Ifit, 'exp1');\ncoeffs=coeffvalues(c);\nIa=coeffs(1);\nRa=dV*1e3./Ia/2;\ntau=-1./coeffs(2);\ncap=tau/Ra*1000;"("data"=w5624, "nsamp"=w5612, "ncyc"=w5616, "maxV"=w5615, "points"=w5622, "srate"=w5614) -> ("cap"=w5611:dbl, "Ra"=w5610:dbl, "Icyc"=w5609:dbl[], "Rm"=w5608:dbl)  [unwired: 1 in, 1 out]
                              n2555 = local read "set as Rp?"() -> (w5623:bool)
                              n2556 = local write "Cmembrane"(w5611) -> ()
                              n2557 = local write "Rmembrane (MOhm)"(w5608) -> ()
                              n2558 = local write "Racces (MOhm)"(w5610) -> ()
                              n2559 = case shown="True" w5623 {
                                tunnel: w5608 -> [_ w5643]
                                frame False {
                                }
                                frame True {
                                n2560 = local write "Rpipette (MOhm)"(w5643) -> ()
                                }
                              }
                              n2561 = local write "Ifit"(w5609) -> ()
                            }
                            frame #5 {
                              n2562 = local read "set as Rp?"() -> (w5645:bool)
                              n2563 = case shown="True" w5644 {
                                frame False {
                                }
                                frame True {
                                n2564 = stacked-sequence {
                                frame #0 {
                                n2565 = call "tempconfigAO.vi"("command"="get") -> ("Temp Config out"=w5652:T25)  [unwired: 1 in]
                                n2566 = Unbundle By Name(w5652) -> ("AO"=w5651:refnum<k21>[], "E_AO"=w5650:errorcluster[])
                                n2567 = for {
                                tunnel: w5651 -> [w5659] mode=indexing
                                tunnel: w5650 -> [w5658] mode=indexing
                                tunnel: [w5657] -> w5648 mode=indexing
                                tunnel: [w5656] -> w5647 mode=indexing
                                n2568 = call <vilib>:"DAQmx Start Task.vi"("task/channels in"=w5659, "error in"=w5658) -> ("task out"=w5657:refnum<k21>, "error out"=w5656:errorcluster)  [unwired: 12 in]
                                }
                                n2569 = call "tempconfigAO.vi"("command"="get") -> ("Temp Config out"=w5649:T25)  [unwired: 1 in]
